vi "SequenceIndicesTCValueChange.vi"(8 "error in (no error)":errorcluster, 10 "ValueChangeIn":T1, 11 "VMUI in":refnum<class "VMUI.lvclass">) -> (0 "error out":errorcluster, 3 "VMUI out":refnum<class "VMUI.lvclass">)   [LabVIEW 2013, in "VMUI.lvclass"]
uses:
  VMUI.lvclass
  API/VariableManagerAPI.lvlib
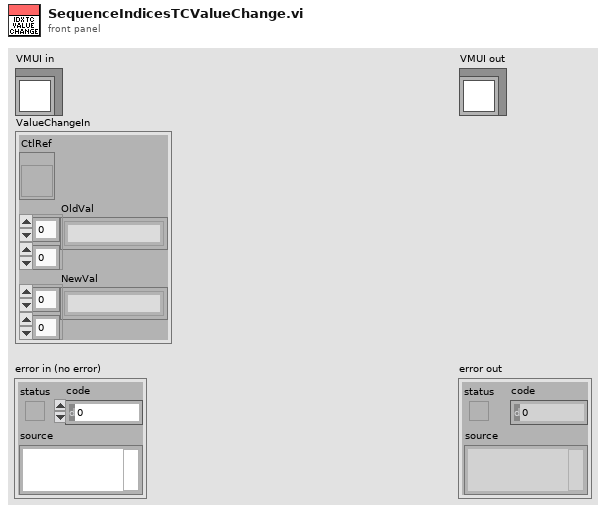
[diagram p1: front panel]
types:
  T1 = cluster{"CtlRef":refnum<vi>, "OldVal":string[][], "NewVal":string[][]}
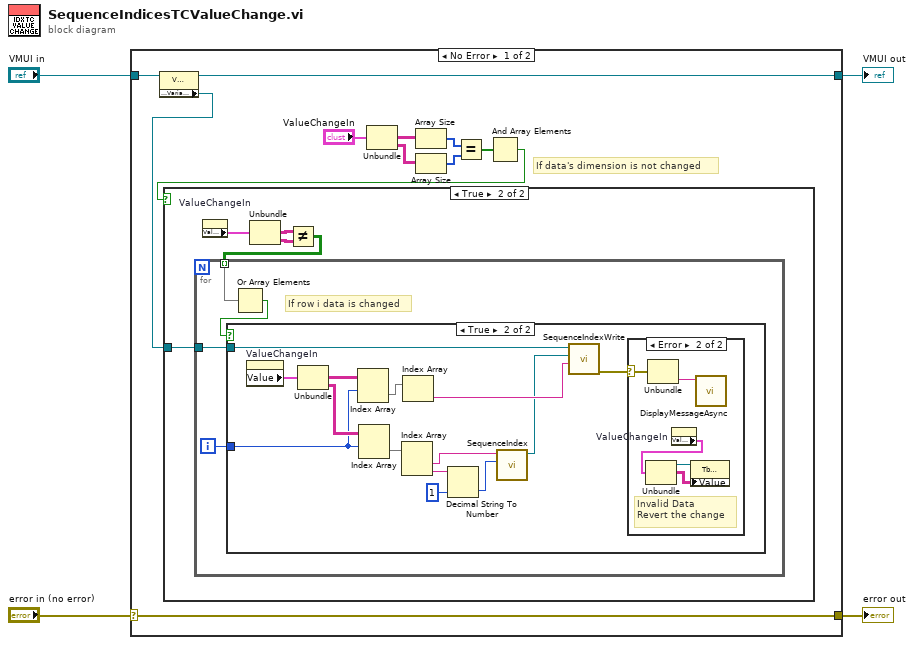
[diagram p0: block diagram]
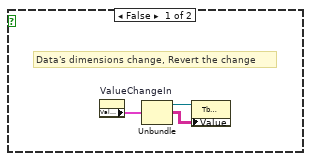
[diagram p2: hidden frame]
diagram:
  n1 = case shown="No Error" "error in (no error)" {
    selector: "error in (no error)" -> [w15 w48]
    tunnel: [w15 w48] -> w3
    tunnel: [w6 w47] -> w1
    tunnel: "VMUI in" -> [w7 w47]
    frame No Error {
      # "If data's dimension is not changed"
      n2 = property class="VMUI.lvclass"(reference=w7) -> (reference out=w6:refnum<class "VMUI.lvclass">, "Accessors:VariableManagerRef"=w5:refnum<vi>)  [unwired: 1 in, 1 out]
      n3 = Unbundle("ValueChangeIn") -> ("OldVal"=w13:string[][], "NewVal"=w14:string[][])  [unwired: 1 out]
      n4 = Array Size(array=w13) -> (size(s)=w8:i32[])
      n5 = Array Size(array=w14) -> (size(s)=w9:i32[])
      n6 = Equal?(x=w8, y=w9) -> (x = y?=w10:bool[])
      n7 = And Array Elements(Boolean array=w10) -> (logical AND=w11:bool)
      n8 = case shown="True" w11 {
        tunnel: w5 -> [_ w19]
        frame False {
          # "Data's dimensions change, Revert the change"
          n9 = property on="ValueChangeIn" class="Clust (strict)"() -> ("Value"=w18:T1)  [unwired: 2 in, 2 out]
          n10 = Unbundle(w18) -> ("CtlRef"=w17:refnum<vi>, "OldVal"=w16:string[][])  [unwired: 1 out]
          n11 = property class="Tbl (strict)"(reference=w17, "Value"=w16) -> ()  [unwired: 1 in, 2 out]
        }
        frame True {
          n12 = property on="ValueChangeIn" class="Clust (strict)"() -> ("Value"=w23:T1)  [unwired: 2 in, 2 out]
          n13 = Unbundle(w23) -> ("OldVal"=w22:string[][], "NewVal"=w21:string[][])  [unwired: 1 out]
          n14 = Not Equal?(x=w22, y=w21) -> (x != y?=w20:bool[][])
          n15 = for {
            tunnel: w20 -> [w27] mode=indexing
            tunnel: w19 -> [w24]
            i -> [w25]
            # "If row i data is changed"
            n16 = Or Array Elements(Boolean array=w27) -> (logical OR=w26:bool)
            n17 = case shown="True" w26 {
              tunnel: w25 -> [_ w37]
              tunnel: w24 -> [_ w33]
              frame False {
                # "No change"
              }
              frame True {
                n18 = property on="ValueChangeIn" class="Clust (strict)"() -> ("Value"=w41:T1)  [unwired: 2 in, 2 out]
                n19 = Unbundle(w41) -> ("OldVal"=w38:string[][], "NewVal"=w40:string[][])  [unwired: 1 out]
                n20 = Index Array(array=w38, index (row)=w37) -> (element=w36:string[])  [unwired: 1 in]
                n21 = Index Array(array=w40, index (row)=w37) -> (element=w39:string[])  [unwired: 1 in]
                n22 = Index Array(array=w39) -> (element #1=w31:string, element #2=w35:string)  [unwired: 2 in]
                n23 = Index Array(array=w36) -> (element=w32:string)  [unwired: 1 in]
                n24 = Decimal String To Number(string=w35, default (0L)=1 ("default (0 I32)")) -> (number=w30:i32)  [unwired: 1 in, 1 out]
                n25 = call "SequenceIndex.vi"("Steps"=w30, "SequenceIndexName"=w31) -> ("SequenceIndex"=w29:refnum<class "SequenceIndex.lvclass">)  [unwired: 9 in]
                n26 = call "SequenceIndexWrite.vi"("OriginalName"=w32, "SequenceIndex"=w29, "VariableManagerRef in"=w33) -> ("error out"=w28:errorcluster)  [unwired: 7 in, 1 out]
                n27 = case shown="Error" w28 {
                  selector: w28 -> [_ w42]
                  frame No Error {
                  }
                  frame Error {
                    # "Invalid Data\nRevert the change"
                    n28 = Unbundle(w42) -> ("source"=w43:string)  [unwired: 2 out]
                    n29 = property on="ValueChangeIn" class="Clust (strict)"() -> ("Value"=w46:T1)  [unwired: 2 in, 2 out]
                    n30 = Unbundle(w46) -> ("CtlRef"=w45:refnum<vi>, "OldVal"=w44:string[][])  [unwired: 1 out]
                    n31 = property class="Tbl (strict)"(reference=w45, "Value"=w44) -> ()  [unwired: 1 in, 2 out]
                    n32 = call "DisplayMessageAsync.vi"("Message"=w43) -> ()  [unwired: 11 in]
                  }
                }
              }
            }
          }
        }
      }
    }
    frame Error {
    }
  }
  "error out" <- w3
  "VMUI out" <- w1
